vi "OE1022D_GPIB_Query Data.vi"(0 "VISA resource name":refnum<visa-resource-name>, 9 "Timeout":u32=1000, 11 "Error in (no error)":errorcluster caption="error out（no error）") -> (4 "VISA resource  out":refnum<visa-resource-name>, 6 "Parameter Values":T1, 8 "Data Array":dbl[](array[numeric]), 10 "Output String":string, 15 "Error out":errorcluster caption="error out")   [LabVIEW 2011]
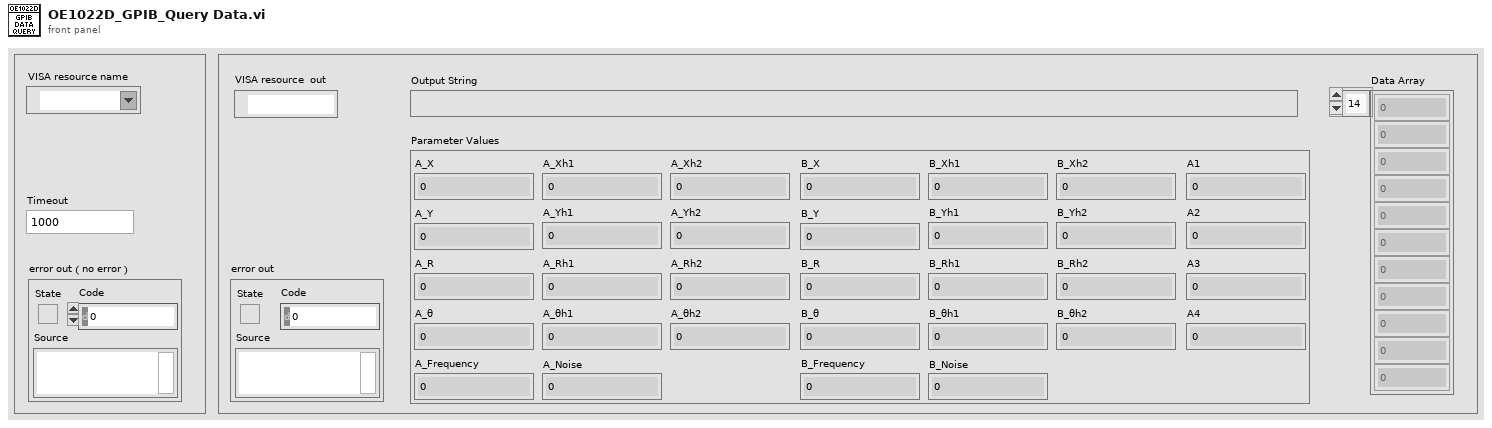
[diagram p1: front panel]
types:
  T1 = cluster{"A_X":dbl, "A_Y":dbl, "A_R":dbl, "A_θ":dbl, "A_Frequency":dbl, "A_Noise":dbl, "A_Xh1":dbl, "A_Yh1":dbl, "A_Rh1":dbl, "A_θh1":dbl, "A_Xh2":dbl, "A_Yh2":dbl, "A_Rh2":dbl, "A_θh2":dbl, "B_X":dbl, "B_Y":dbl, "B_R":dbl, "B_θ":dbl, "B_Frequency":dbl, "B_Noise":dbl, "B_Xh1":dbl, "B_Yh1":dbl, "B_Rh1":dbl, "B_θh1":dbl, "B_Xh2":dbl, "B_Yh2":dbl, "B_Rh2":dbl, "B_θh2":dbl, "A1":dbl, "A2":dbl, "A3":dbl, "A4":dbl}
  T2 = enum16{"ISRC", "IGND", "ICPL", "ILIN", "PHAS", "FMOD", "RSLP", "FREQ", "SWPT", "SLLM", "SULM", "SSLL", "SSLG", "STLM", "SWRM", "IRNG", "SENS", "RMOD", "OFLT", "OFSL", "SYNC", "DMOD", "HARM", "DARB", "SWVT", "SLVL", "SVLL", "SVUL", "SVSL", "SVSG", "SVTM", "SVRM", "RALL", "SNAP", "OUTP", "OAUX", "COUT", "CAUX", "COFP", "CEXP", "FPOP", "OEXP", "*IDN", "*RST", "OVLD", "INOV", "GNOV", "*PLL", "SSET", "RSET", "AGAN", "APHS", "ARSV", "ASCL", "EQCD", "EQCS", "SPED", "SRAT", "SLEN", "SSLE", "STRG", "SPRM", "STRD", "PAUS", "REST", "SPTS", "TRCA", "TEMP", "RSTU", "IHNZ", "DEQU", "SADD", "ARNG", "CSPE", "ISRCD", "IGNDD", "ICPLD", "ILIND", "PHASD", "FMODD", "RSLPD", "FREQD", "SWPTD", "SLLMD", "SULMD", "SSLLD", "SSLGD", "STLMD", "SWRMD", "SENSD", "RMODD", "OFLTD", "OFSLD", "SYNCD", "HARMD", "EQCDD", "EQCSD", "SNAPD", "OUTPD", "SWVTD", "SLVLD", "SVLLD", "SVULD", "SVSLD", "SVSGD", "SVTMD", "SVRMD", "SVDCD", "ARSVD", "AGAND", "APHSD", "ASCLD", "FPOPD", "CAUXD", "OEXPD", "SPEDD", "SRATD", "SLEND", "SSLED", "STRGD", "SPRMD", "STRDD", "PAUSD", "RESTD", "SPTSD", "TRCAD", "*IDND", "*RSTD", "INOVD", "GNOVD", "*PLLD", "SSETD", "RSETD", "RALLD"}
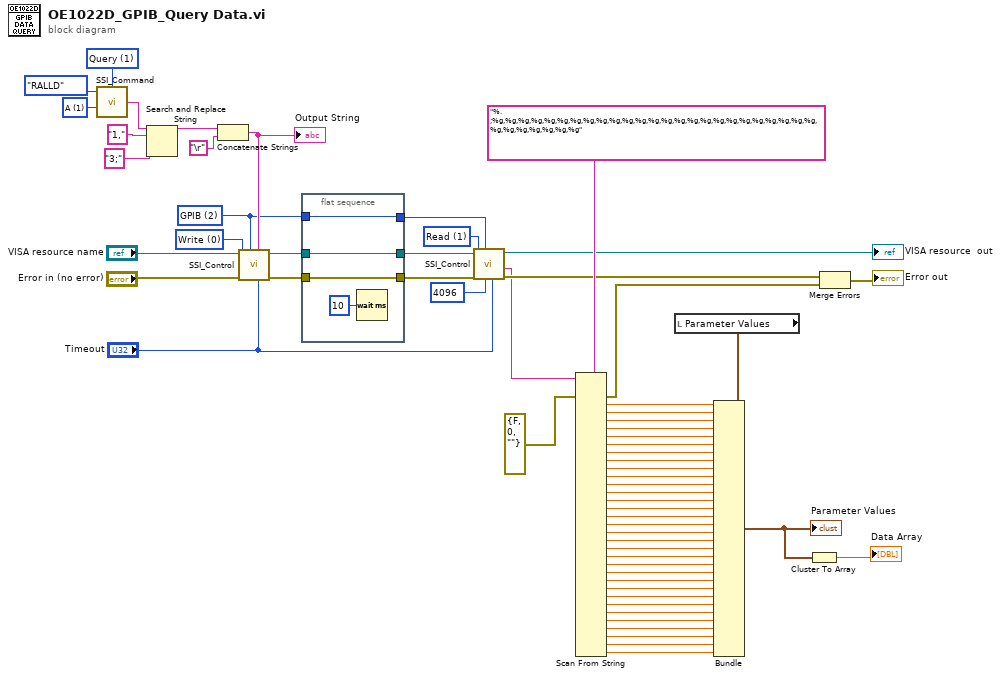
[diagram p0: block diagram]
diagram:
  w3 = u16 1 items=["A"=1, "B"=2, "None"=0] ("channel")
  w50 = u16 1 items=["Set", "Query"] ("Opera")
  w53 = u16 2 items=["USB", "RS232", "GPIB", "Ethernet"] ("Remote Mode")
  w56 = u16 1 items=["Write", "Read"] ("Control")
  w61 = u16 0 items=["Write", "Read"] ("Control")
  n1 = call "SSI_Command.vi"("Opera"=w50, "channel"=w3, "Command Type"=T2."RALLD") -> ("Output string"=w5:string)  [unwired: 1 in]
  n2 = Search and Replace String(input string=w5, search string="1," ("搜索字符串"), replace string="3;" ("替换字符串(\"\")")) -> (result string=w2:string)  [unwired: 5 in, 3 out]
  n3 = Concatenate Strings(w2, "\r") -> (w54:string)
  "Output String" <- w54
  n4 = call "SSI_Control.vi"("Tineout"="Timeout", "Write Buffer"=w54, "Remote Mode"=w53, "Error in (no error)"="Error in (no error)", "Control"=w61, "VISA resource name"="VISA resource name") -> ("Error out"=w59:errorcluster, "VISA resource  out"=w60:refnum<visa-resource-name>)  [unwired: 2 in, 2 out]
  n5 = flat-sequence {
    tunnel: w60 -> [w67]
    tunnel: w59 -> [w66]
    tunnel: [w67] -> w58
    tunnel: [w66] -> w57
    tunnel: [w64] -> w28
    tunnel: w53 -> [w64]
    frame #0 {
      n6 = Wait (ms)(milliseconds to wait=u32 10 ("等待时间（毫秒）")) -> ()  [unwired: 1 out]
    }
  }
  n7 = call "SSI_Control.vi"("Tineout"="Timeout", "Number of bytes"=u32 4096, "Remote Mode"=w28, "Error in (no error)"=w57, "Control"=w56, "VISA resource name"=w58) -> ("Error out"=w27:errorcluster, "Read Buffer"=w7:string, "VISA resource  out"=→"VISA resource  out":refnum<visa-resource-name>)  [unwired: 2 in, 1 out]
  n8 = Scan From String(format string="%.;%g,%g,%g,%g,%g,%g,%g,%g,%g,%g,%g,%g,%g,%g,%g,%g,%g,%g,%g,%g,%g,%g,%g,%g,%g,%g,%g,%g,%g,%g,%g,%g" ("格式字符串"), input string=w7, error in=errorcluster {"status"=FALSE, "code"=0, "source"=""} ("error constant")) -> (error out=w6:errorcluster, output 1=w35:dbl, output 2=w34:dbl, output 3=w37:dbl, output 4=w38:dbl, output 5=w39:dbl, output 6=w40:dbl, output 7=w41:dbl, output 8=w42:dbl, output 9=w43:dbl, output 10=w44:dbl, output 11=w45:dbl, output 12=w46:dbl, output 13=w47:dbl, output 14=w48:dbl, output 15=w25:dbl, output 16=w24:dbl, output 17=w23:dbl, output 18=w22:dbl, output 19=w21:dbl, output 20=w20:dbl, output 21=w19:dbl, output 22=w17:dbl, output 23=w18:dbl, output 24=w16:dbl, output 25=w14:dbl, output 26=w15:dbl, output 27=w13:dbl, output 28=w12:dbl, output 29=w11:dbl, output 30=w10:dbl, output 31=w9:dbl, output 32=w8:dbl)  [unwired: 33 in, 2 out]
  n9 = local read "Parameter Values"() -> (w36:T1)
  n10 = Bundle(cluster=w36, "A_X"=w35, "A_Y"=w34, "A_R"=w37, "A_θ"=w38, "A_Frequency"=w39, "A_Noise"=w40, "A_Xh1"=w41, "A_Yh1"=w42, "A_Rh1"=w43, "A_θh1"=w44, "A_Xh2"=w45, "A_Yh2"=w46, "A_Rh2"=w47, "A_θh2"=w48, "B_X"=w25, "B_Y"=w24, "B_R"=w23, "B_θ"=w22, "B_Frequency"=w21, "B_Noise"=w20, "B_Xh1"=w19, "B_Yh1"=w17, "B_Rh1"=w18, "B_θh1"=w16, "B_Xh2"=w14, "B_Yh2"=w15, "B_Rh2"=w13, "B_θh2"=w12, "A1"=w11, "A2"=w10, "A3"=w9, "A4"=w8) -> (w32:T1)
  "Parameter Values" <- w32
  n11 = Cluster To Array(cluster=w32) -> (array=→"Data Array":dbl[])
  n12 = Merge Errors(w27, w6) -> (→"Error out":errorcluster)
